vi "myRIO_BRig Encoder Store Overflow.vi"(7 "Clear?":bool, 11 "Over?":bool) -> (2 "Error?":bool, 3 "Overflow?":bool)   [LabVIEW 2014]
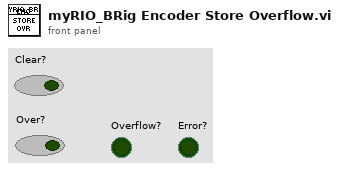
[diagram p1: front panel]
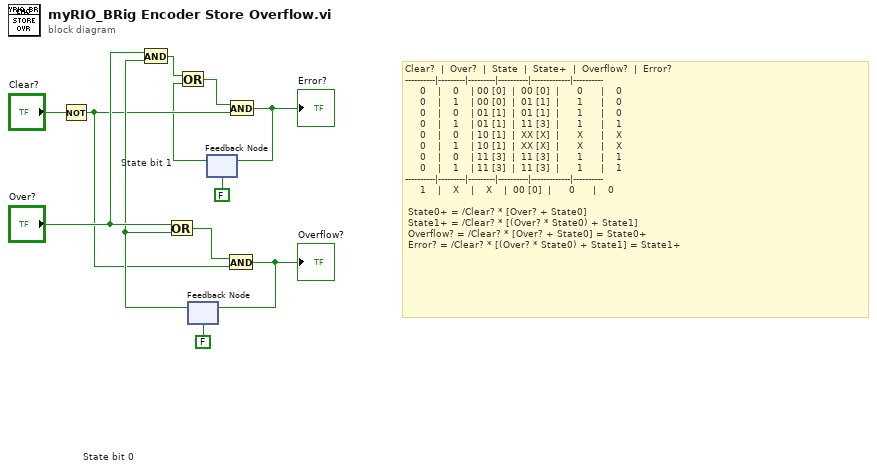
[diagram p0: block diagram]
diagram:
  # "Clear?  |  Over?  |  State  |  State+  |  Overflow?  |  Error?  \n----------|---------|---------|----------|-------------|----------\n     0    |    0    | 00 [0]  |  00 [0]  |      0      |    0\n     0    |    1    | 00 [0]  |  01 [1]  |      1      |    0\n     0    |    0    | 01 [1]  |  01 [1]  |      1      |    0\n     0    |    1    | 01 [1]  |  11 [3]  |      1      |    1\n     0    |    0    | 10 [1]  |  XX [X]  |      X      |    X\n     0    |    1    | 10 [1]  |  XX [X]  |      X      |    X\n     0    |    0    | 11 [3]  |  11 [3]  |      1      |    1\n     0    |    1    | 11 [3]  |  11 [3]  |      1      |    1\n----------|---------|---------|----------|-------------|----------\n     1    |    X    |    X    |  00 [0]  |      0      |    0\n\n State0+ = /Clear? * [Over? + State0]\n State1+ = /Clear? * [(Over? * State0) + State1]\n Overflow? = /Clear? * [Over? + State0] = State0+\n Error? = /Clear? * [(Over? * State0) + State1] = State1+"
  n1 = Not(x="Clear?") -> (.not. x?=w4:bool)
  n2 = feedback #1 "State bit 0"(FALSE) -> (w5:bool)
  n3 = And(x="Over?", y=w5) -> (x .and. y?=w3:bool)
  n4 = Or(x="Over?", y=w5) -> (x .or. y?=w11:bool)
  n5 = feedback #2 "State bit 1"(FALSE) -> (w2:bool)
  n6 = Or(x=w3, y=w2) -> (x .or. y?=w1:bool)
  n7 = And(x=w11, y=w4) -> (x .and. y?=w10:bool)
  "Overflow?" <- w10
  n8 = feedback-in #1(w10) -> ()
  n9 = And(x=w1, y=w4) -> (x .and. y?=w8:bool)
  "Error?" <- w8
  n10 = feedback-in #2(w8) -> ()
